vi "Copy Create Dirs.vi"(8 "Error In":errorcluster, 10 "Destination":path, 11 "Source":path) -> (0 "Error Out":errorcluster)   [LabVIEW 2011, in "LVH-LINX.lvlib"]
doc: "Copy a file and create destination directory hierarchy if necissary."
uses:
  LVH-LINX.lvlib
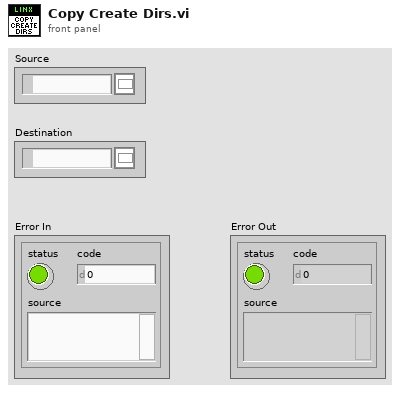
[diagram p1: front panel]
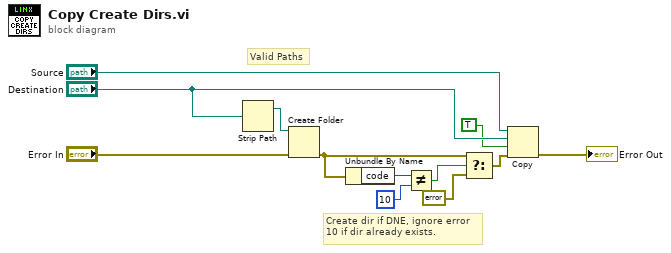
[diagram p0: block diagram]
diagram:
  # "Valid Paths"
  # "Create dir if DNE, ignore error\n10 if dir already exists."
  n1 = Strip Path(path="Destination") -> (stripped path=w7:path)  [unwired: 1 out]
  n2 = Create Folder(path (use dialog)=w7, error in="Error In") -> (error out=w4:errorcluster)  [unwired: 1 in, 2 out]
  n3 = Unbundle By Name(w4) -> ("code"=w6:i32)
  n4 = Not Equal?(x=w6, y=10) -> (x != y?=w3:bool)
  n5 = Select(t=w4, s=w3, f=errorcluster {"status"=FALSE, "code"=0, "source"=""}) -> (s? t:f=w1:errorcluster)
  n6 = Copy(8:w1, 9:TRUE ("overwrite (F)"), 10:"Destination", 11:"Source") -> (0:→"Error Out":errorcluster)  [unwired: 1 in, 2 out]
